vi "ziGetValueDemodSampleEx.vi"(3 "error in":errorcluster, 4 "Path":string, 5 "Handle In":T2 {"Handle" format="0x%08x"; "Conn" format="0x%08x"}) -> (0 "error out":errorcluster, 1 "Demod Sample Out":T1={"Timestamps (ticks)"=0, "X (Vrms)"=nan, "Y (Vrms)"=nan, "Osc Phase (deg)"=nan, "Freq (Hz)"=nan, "DIO"=0, "AuxIn0 (V)"=nan, "AuxIn1 (V)"=nan, "Trigger"=0}, 2 "Handle Out":T2 {"Handle" format="0x%08x"; "Conn" format="0x%08x"})   [LabVIEW 2018, in "Zurich Instruments LabOne.lvlib"]
doc: "This function retrieves the newest available sample from a demodulator's sample node. The value first found is returned if more than one value is available (a wildcard is used in the path). This function is only applicable to paths matching DEMODS/[0-9]+/SAMPLE."
uses:
  Zurich Instruments LabOne.lvlib
  <instrlib>/Zurich Instruments LabOne/Private/ziLV64.framework
  Data/ziTypeDemodSampleSingle.ctl
  ziTypeHandle.ctl
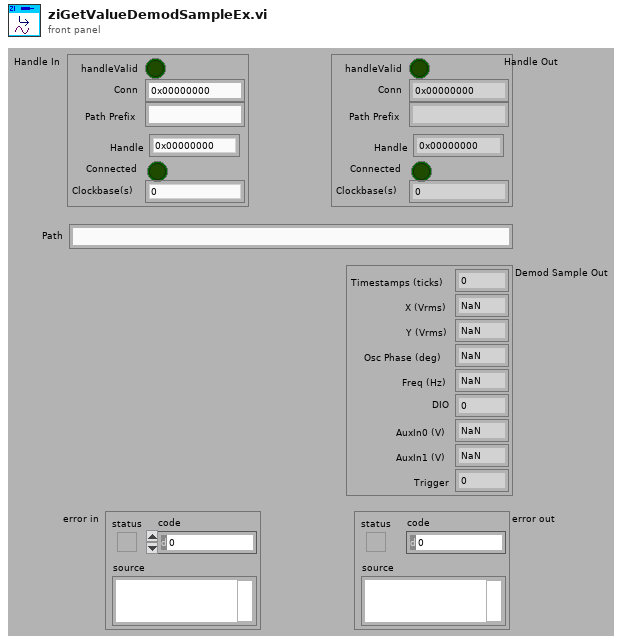
[diagram p1: front panel]
types:
  T1 = typedef "Zurich Instruments LabOne.lvlib/ziTypeDemodSampleSingle.ctl" = cluster{"Timestamps (ticks)":u64, "X (Vrms)":dbl, "Y (Vrms)":dbl, "Osc Phase (deg)":dbl, "Freq (Hz)":dbl, "DIO":u32, "AuxIn0 (V)":dbl, "AuxIn1 (V)":dbl, "Trigger":u32}
  T2 = typedef "Zurich Instruments LabOne.lvlib/ziTypeHandle.ctl" = cluster{"handleValid":bool, "Conn":u64, "Path Prefix":string, "Handle":u64, "Connected":bool, "Clockbase(s)":dbl}
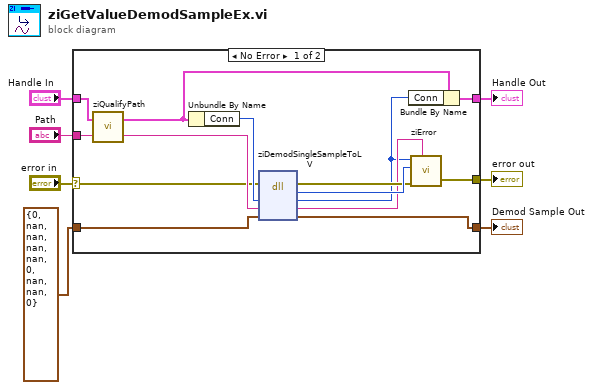
[diagram p0: block diagram]
diagram:
  n1 = case shown="No Error" "error in" {
    selector: "error in" -> [w11 w23]
    tunnel: [w9 w23] -> w7
    tunnel: [w18 w24] -> w6
    tunnel: "Path" -> [w17 _]
    tunnel: "Handle In" -> [w15 w24]
    tunnel: [w8 w22] -> w1
    tunnel: T1 {"Timestamps (ticks)"=0, "X (Vrms)"=nan, "Y (Vrms)"=nan, "Osc Phase (deg)"=nan, "Freq (Hz)"=nan, "DIO"=0, "AuxIn0 (V)"=nan, "AuxIn1 (V)"=nan, "Trigger"=0} ("Demod Sample Out") -> [w10 w22]
    frame No Error {
      n2 = call "ziQualifyPath.vi"("Path In"=w17, "Handle In"=w15) -> ("Path Out"=w16:string, "Handle Out"=w14:T2)
      n3 = Unbundle By Name(w14) -> ("Conn"=w21:u64)
      n4 = dll-call lib="Applications/National Instruments/LabVIEW 2019 64-bit/instr.lib/Zurich Instruments LabOne/Private/ziLV*.*" fn="ziDemodSingleSampleToLV" label="ziAPIGetDemodSample"(error in=w11, "Conn"=w21, "Path"=w16, w10) -> (error out=w19:errorcluster, "return type"=w20:u32, "Conn"=w12:u64, "Path"=w13:string, w8:T1)  [unwired: 2 in, 1 out]
      n5 = Bundle By Name(cluster=w14, "Conn"=w12) -> (w18:T2)
      n6 = call "ziError.vi"("Conn"=w12, "ziErrorCode"=w20, "Error In"=w19, "Annotation"=w13) -> ("Error Out"=w9:errorcluster)  [unwired: 1 in, 1 out]
    }
    frame Error {
    }
  }
  "Handle Out" <- w6
  "error out" <- w7
  "Demod Sample Out" <- w1
